vi "set task timing.vi"(8 "error in (no error)":errorcluster, 11 "Waveform in":refnum<class "Waveform.lvclass">) -> (0 "error out":errorcluster, 3 "Waveform out":refnum<class "Waveform.lvclass">)   [LabVIEW 2012, in "Waveform.lvclass"]
uses:
  Waveform.lvclass
  Waveform.lvclass/Waveform.ctl
  <vilib>/DAQmx/configure/timing.llb/DAQmx Timing (Implicit).vi
  <vilib>/DAQmx/configure/timing.llb/DAQmx Timing (Sample Clock).vi
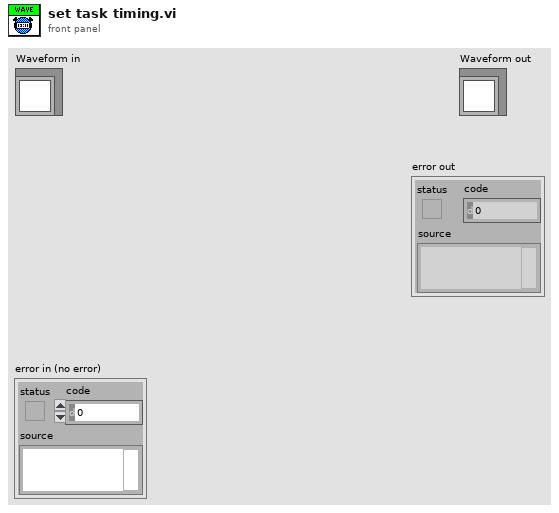
[diagram p1: front panel]
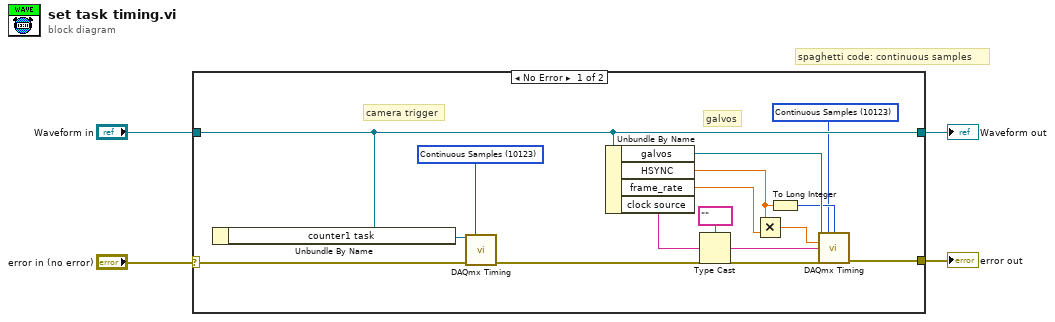
[diagram p0: block diagram]
diagram:
  # "spaghetti code: continuous samples"
  n1 = case shown="No Error" "error in (no error)" {
    selector: "error in (no error)" -> [w17 w21]
    tunnel: [w6 w21] -> w3
    tunnel: [w14 w20] -> w1
    tunnel: "Waveform in" -> [w14 w20]
    frame No Error {
      w11 = 10123 items=["Finite Samples"=10178, "Continuous Samples"=10123, "Hardware Timed Single Point"=12522] ("sample mode")
      w19 = 10123 items=["Finite Samples"=10178, "Continuous Samples"=10123, "Hardware Timed Single Point"=12522] ("sample mode")
      # "galvos"
      # "camera trigger"
      n2 = Unbundle By Name(w14) -> ("counter1 task"=w18:refnum<k21>)
      n3 = call-poly <vilib>:"DAQmx Timing.vi"("task/channels in"=w18, "sample mode"=w19, "error in"=w17) -> ("error out"=w9:errorcluster)  [unwired: 11 in, 1 out]
      n4 = Unbundle By Name(w14) -> ("galvos"=w13:refnum<k21>, "HSYNC"=w15:dbl, "frame_rate"=w16:dbl, "clock source"=w8:string)
      n5 = Type Cast(type=tag "" ("source"), x=w8) -> (*(type *) &x=w5:tag)
      n6 = Multiply(x=w15, y=w16) -> (x*y=w10:dbl)
      n7 = To Long Integer(number=w15) -> (32bit integer=w12:i32)
      n8 = call-poly <vilib>:"DAQmx Timing.vi"("task/channels in"=w13, "sample mode"=w11, "samples per channel"=w12, "rate"=w10, "source"=w5, "error in"=w9) -> ("error out"=w6:errorcluster)  [unwired: 8 in, 1 out]
    }
    frame Error {
    }
  }
  "error out" <- w3
  "Waveform out" <- w1
